vi "createM1M3SAL.vi"(8 "error in (no error)":errorcluster, 11 "Boot in":refnum<class "Boot.lvclass">) -> (0 "error out":errorcluster, 2 "M1M3SAL":refnum<class "M1M3SAL.lvclass">, 3 "Boot out":refnum<class "Boot.lvclass">)   [LabVIEW 2016, in "Boot.lvclass"]
uses:
  Boot.lvclass
  Communicator/M1M3SAL/M1M3SAL.lvclass
  Communicator/M1M3SAL/M1M3SAL.lvclass/M1M3SAL.ctl
  Boot.lvclass/Boot.ctl
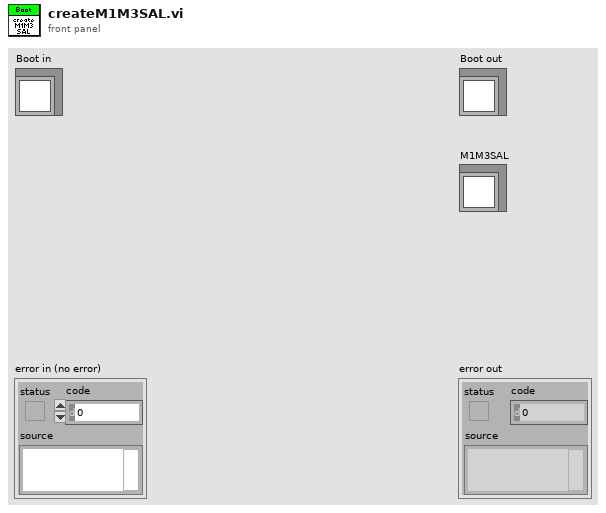
[diagram p1: front panel]
types:
  T1 = typedef "M1M3SupportSettings.lvlib/BaseSALSettings.ctl" = cluster{"Connection":T2}
  T2 = typedef "M1M3SupportCommunicator.lvlib/M1M3SALSettings.ctl" = cluster{"IPAddress":string, "Port":u16, "StartupScript":string}
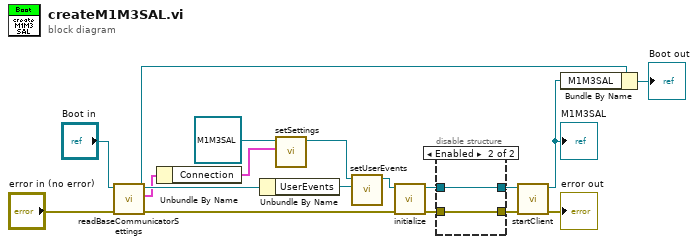
[diagram p0: block diagram]
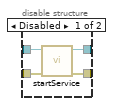
[diagram p2: hidden frame]
diagram:
  n1 = call "readBaseCommunicatorSettings.vi"("error in (no error)"="error in (no error)", "Boot in"="Boot in") -> ("error out"=w2:errorcluster, "M1M3SALSettings"=w6:T1, "Boot out"=w11:refnum<class "Boot.lvclass">)  [unwired: 7 in]
  n2 = Unbundle By Name(w6) -> ("Connection"=w5:T2)
  n3 = Unbundle By Name(w11) -> ("UserEvents"=w13:refnum<class "UserEvents.lvclass">)
  n4 = call "setSettings.vi"("Settings"=w5, "M1M3SAL in"=refnum<class "M1M3SAL.lvclass"> refnum ("M1M3Communicator.lvlib:M1M3SAL.lvclass")) -> ("M1M3SAL out"=w16:refnum<class "M1M3SAL.lvclass">)  [unwired: 9 in]
  n5 = call "setUserEvents.vi"("UserEvents"=w13, "M1M3SAL in"=w16) -> ("M1M3SAL out"=w4:refnum<class "M1M3SAL.lvclass">)  [unwired: 9 in]
  n6 = call "initialize.vi"("error in (no error)"=w2, "M1M3SAL in"=w4) -> ("error out"=w1:errorcluster, "M1M3SAL out"=w3:refnum<class "M1M3SAL.lvclass">)  [unwired: 8 in]
  n7 = disable-structure shown="Enabled" {
    disable-tunnel: w3 -> [w21 w23]
    disable-tunnel: [w20 w23] -> w15
    disable-tunnel: [w19 w22] -> w14
    disable-tunnel: w1 -> [w18 w22]
    frame Disabled {
      n8 = call "startService.vi"("error in (no error)"=w18, "M1M3SAL in"=w21) -> ("error out"=w19:errorcluster, "M1M3SAL out"=w20:refnum<class "M1M3SAL.lvclass">)  [unwired: 8 in]
    }
    frame Enabled {
    }
  }
  n9 = call "startClient.vi"("error in (no error)"=w14, "M1M3SAL in"=w15) -> ("error out"=→"error out":errorcluster, "M1M3SAL out"=w9:refnum<class "M1M3SAL.lvclass">)  [unwired: 8 in]
  "M1M3SAL" <- w9
  n10 = Bundle By Name(cluster=w11, "M1M3SAL"=w9) -> (→"Boot out":refnum<class "Boot.lvclass">)
